vi "Create CPU Bar.vi"(8 "error in (no error)":errorcluster, 9 "CPU Info":cluster{"CPU Index":i32, "# of CPUs":i32}, 10 "Draw Area Size":T1) -> (0 "error out":errorcluster, 3 "Shape Reference":refnum<data-value>)   [LabVIEW 2016, in "CPU Bar.lvclass"]
uses:
  CPU Bar.lvclass
  <vilib>/LIEF/Forms/Shape/Shape.lvclass
  <vilib>/Utility/miscctls.llb/LVBoundsTypeDef.ctl
  C:/Program Files (x86)/National Instruments/LabVIEW 2016/vi.lib/LIEF/Forms/Layered Shape/Layered Shape.lvclass
  C:/Program Files (x86)/National Instruments/LabVIEW 2016/vi.lib/LIEF/Forms/Shape/Shape.lvclass
  C:/Program Files (x86)/National Instruments/LabVIEW 2016/vi.lib/LIEF/Forms/Rectangle/Rectangle.lvclass
  <vilib>/LIEF/Forms/Text/Text.lvclass
  <vilib>/LIEF/Forms/Shape/Shape.lvclass/Shape.ctl
  <vilib>/LIEF/Forms/Rectangle/Rectangle.lvclass/Rectangle.ctl
  <vilib>/LIEF/Forms/Layered Shape/Layered Shape.lvclass/Layered Shape.ctl
  <vilib>/LIEF/Forms/Shape/Write Color.vi
  <vilib>/LIEF/Forms/Rectangle/Write Filled.vi
  <vilib>/LIEF/Forms/Shape/Write Movable.vi
  <vilib>/LIEF/Forms/Layered Shape/Write Overlays.vi
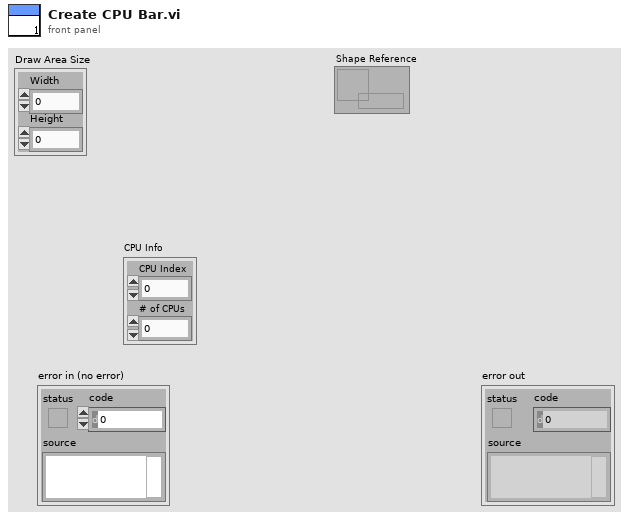
[diagram p1: front panel]
types:
  T1 = typedef "LVBoundsTypeDef.ctl" = cluster{"Width":u32, "Height":u32}
  T2 = cluster{"Font Name:":string, "Size":i16, "Strikeout?":bool, "Italic?":bool, "Underline?":bool, "Outline?":bool, "Shadow?":bool, "Bold?":bool}
  T3 = enum16{"Left", "Top", "Right", "Bottom", "Centered"}
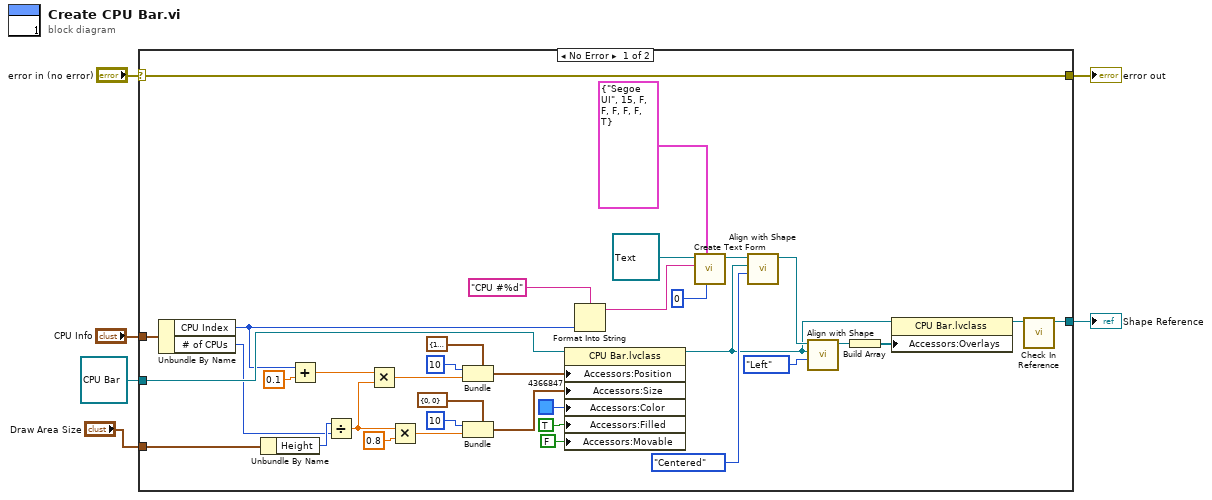
[diagram p0: block diagram]
diagram:
  n1 = case shown="No Error" "error in (no error)" {
    selector: "error in (no error)" -> [w42 w43]
    tunnel: [w42 w43] -> w5
    tunnel: refnum<class "CPU Bar.lvclass"> refnum ("CPU Bar in") -> [w41 _]
    tunnel: "CPU Info" -> [w40 _]
    tunnel: [w18 _] -> w2
    tunnel: "Draw Area Size" -> [w8 _]
    frame No Error {
      n2 = Unbundle By Name(w40) -> ("CPU Index"=w23:i32, "# of CPUs"=w33:i32)
      n3 = Unbundle By Name(w8) -> ("Height"=w39:u32)
      n4 = Add(x=w23, y=0.1) -> (x+y=w32:dbl)
      n5 = Divide(x=w39, y=w33) -> (x/y=w34:dbl)
      n6 = Multiply(x=w32, y=w34) -> (x*y=w30:dbl)
      n7 = Multiply(x=w34, y=0.8) -> (x*y=w36:dbl)
      n8 = Bundle(cluster=cluster{"Left":i32, "Top":i32} {"Left"=10, "Top"=0} ("Position"), "Left"=10, "Top"=w30) -> (w28:cluster{"Left":i32, "Top":i32})
      n9 = Bundle(cluster=cluster{"Width":i32, "Height":i32} {"Width"=0, "Height"=0} ("Size"), "Width"=10, "Height"=w36) -> (w26:cluster{"Width":i32, "Height":i32})
      n10 = property class="CPU Bar.lvclass"(reference=w41, "Accessors:Position"=w28, "Accessors:Size"=w26, "Accessors:Color"=u32 4366847, "Accessors:Filled"=TRUE ("Filled"), "Accessors:Movable"=FALSE ("Movable")) -> (reference out=w15:refnum<class "CPU Bar.lvclass">)  [unwired: 1 in, 1 out]
      n11 = Format Into String(format string="CPU #%d", w23) -> (resulting string=w12:string)  [unwired: 2 in, 1 out]
      n12 = call <vilib>:"Create Text Form.vi"("Color"=u32 0, "[user-specified font]"=T2 {"Font Name:"="Segoe UI", "Size"=15, "Strikeout?"=FALSE, "Italic?"=FALSE, "Underline?"=FALSE, "Outline?"=FALSE, "Shadow?"=FALSE, "Bold?"=TRUE}, "Text"=w12, "Text in"=refnum<class "Text.lvclass"> refnum ("LV Image Editor Framework.lvlib:Text.lvclass")) -> ("New Text"=w11:refnum<class "Text.lvclass">)  [unwired: 6 in, 1 out]
      n13 = call <vilib>:"Align with Shape.vi"("Alignment"=T3."Centered", "Reference Shape"=w15, "Shape in"=w11) -> ("Shape out"=w17:refnum<class "Text.lvclass">)  [unwired: 7 in, 1 out]
      n14 = call <vilib>:"Align with Shape.vi"("Alignment"=T3."Left", "Reference Shape"=w15, "Shape in"=w17) -> ("Shape out"=w16:refnum<class "Text.lvclass">)  [unwired: 7 in, 1 out]
      n15 = Build Array(w16) -> (w20:refnum<class "Text.lvclass">[])
      n16 = property class="CPU Bar.lvclass"(reference=w15, "Accessors:Overlays"=w20) -> (reference out=w19:refnum<class "CPU Bar.lvclass">)  [unwired: 1 in, 1 out]
      n17 = call <vilib>:"Check In Reference.vi"("Shape in"=w19) -> ("Shape Reference"=w18:refnum<data-value>)  [unwired: 9 in, 1 out]
    }
    frame Error {
    }
  }
  "error out" <- w5
  "Shape Reference" <- w2
